vi "Find Appropriate Subsequences for Cx.vi"(10 "All Subarrays Out 2":T1[](array[typedef]), 11 "All Subarrays Out 1":T1[](array[typedef])) -> (3 "Appropriate Subsequences":T2[](array[typedef]))   [LabVIEW 2013, in "GA.lvclass"]
uses:
  GA.lvclass
  Controls/Appropraite Subsequences for SXX.ctl
  Controls/Subsequence.ctl
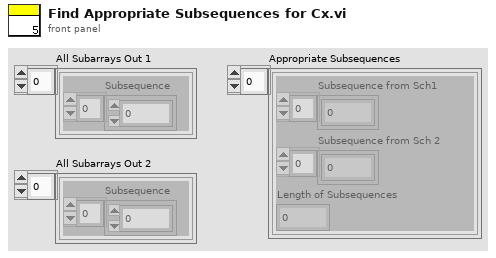
[diagram p1: front panel]
types:
  T1 = typedef "Subsequence.ctl" = cluster{"Subsequence":i32[]}
  T2 = typedef "Appropraite Subsequences for SXX.ctl" = cluster{"Subsequence from Sch1":i32[], "Subsequence from Sch 2":i32[], "Length of Subsequences":i32}
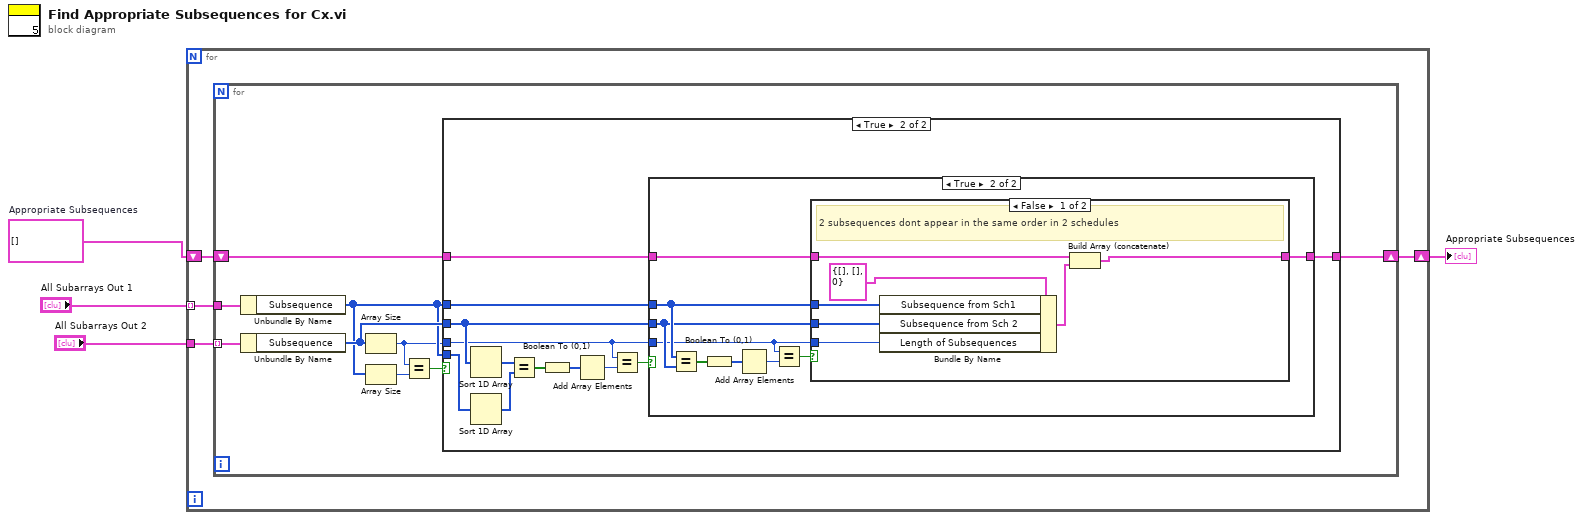
[diagram p0: block diagram]
diagram:
  w1 = T2[] []  # Appropriate Subsequences
  n1 = for {
    tunnel: "All Subarrays Out 1" -> [w7] mode=indexing
    tunnel: "All Subarrays Out 2" -> [w8]
    shift-right: [w5] -> w4
    shift-left: w1 -> [w6]
    n2 = for {
      tunnel: w8 -> [w16] mode=indexing
      tunnel: w7 -> [w17]
      shift-right: [w9] -> w5
      shift-left: w6 -> [w12]
      n3 = Unbundle By Name(w17) -> ("Subsequence"=w11:i32[])
      n4 = Unbundle By Name(w16) -> ("Subsequence"=w13:i32[])
      n5 = Array Size(array=w13) -> (size(s)=w10:i32)
      n6 = Array Size(array=w11) -> (size(s)=w15:i32)
      n7 = Equal?(x=w10, y=w15) -> (x = y?=w14:bool)
      n8 = case shown="True" w14 {
        tunnel: w13 -> [_ w27]
        tunnel: w11 -> [_ w30]
        tunnel: w12 -> [w18 w26]
        tunnel: w11 -> [_ w28]
        tunnel: w10 -> [_ w19]
        tunnel: [w18 w25] -> w9
        frame False {
        }
        frame True {
          n9 = Sort 1D Array(array=w27) -> (sorted array=w23:i32[])
          n10 = Sort 1D Array(array=w30) -> (sorted array=w22:i32[])
          n11 = Equal?(x=w23, y=w22) -> (x = y?=w21:bool[])
          n12 = Boolean To (0,1)(Boolean=w21) -> (0, 1=w20:i16[])
          n13 = Add Array Elements(numeric array=w20) -> (sum=w29:i16)
          n14 = Equal?(x=w19, y=w29) -> (x = y?=w24:bool)
          n15 = case shown="True" w24 {
            tunnel: w28 -> [_ w36]
            tunnel: w27 -> [_ w35]
            tunnel: w19 -> [_ w32]
            tunnel: w26 -> [w31 w40]
            tunnel: [w31 w39] -> w25
            frame False {
            }
            frame True {
              n16 = Equal?(x=w36, y=w35) -> (x = y?=w34:bool[])
              n17 = Boolean To (0,1)(Boolean=w34) -> (0, 1=w33:i16[])
              n18 = Add Array Elements(numeric array=w33) -> (sum=w38:i16)
              n19 = Equal?(x=w32, y=w38) -> (x = y?=w37:bool)
              n20 = case shown="False" w37 {
                tunnel: w32 -> [w46 _]
                tunnel: w40 -> [w45 w48]
                tunnel: [w43 w48] -> w39
                tunnel: w36 -> [w42 _]
                tunnel: w35 -> [w41 _]
                frame False {
                  # "2 subsequences dont appear in the same order in 2 schedules"
                  n21 = Bundle By Name(cluster=T2 {"Subsequence from Sch1"=[], "Subsequence from Sch 2"=[], "Length of Subsequences"=0}, "Subsequence from Sch1"=w42, "Subsequence from Sch 2"=w41, "Length of Subsequences"=w46) -> (w44:T2)
                  n22 = Build Array (concatenate)(w45, w44) -> (w43:T2[])
                }
                frame True {
                  # "2 subsequences appear in the same order in 2 schedules"
                }
              }
            }
          }
        }
      }
    }
  }
  "Appropriate Subsequences" <- w4
